vi "Instrument Locations.vi"() -> ()   [LabVIEW 2016, in "Hall Effect Library.lvlib"]
uses:
  Hall Effect Library.lvlib
panel:
  in  "Magnet":refnum<visa-resource-name>
  in  "Ammeter":refnum<visa-resource-name>
  in  "Switch":refnum<visa-resource-name>
  in  "V-Meter":refnum<visa-resource-name>
  in  "I-SRC":refnum<visa-resource-name>
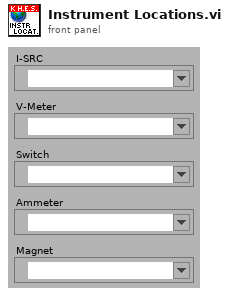
[diagram p1: front panel]
diagram:
